vi "test_GetName.vi"() -> ()   [LabVIEW 2013]
uses:
  <vilib>/Utility/GetType.llb/Type Enum.ctl
  source/TypeDescriptor/TypeDescriptor_GetPString.vi
panel:
  out "Renamed Successfully":bool
  out "type descriptor dup 2":i16[](array[numeric]) format="%.0x"
  out "Type Enum 2":T1=enum."String"
  out "data string":string
  out "name":string
  out "interleaved array":u8[](array[numeric]) format="%.0x"
  out "type descriptor dup":i16[](array[numeric])
  # "index 2 = nb elements"
  # "size = 10 (xA)"
  # "Event DataType (x3 = I32)"
  # "size"
  # "TypeLabel (test)"
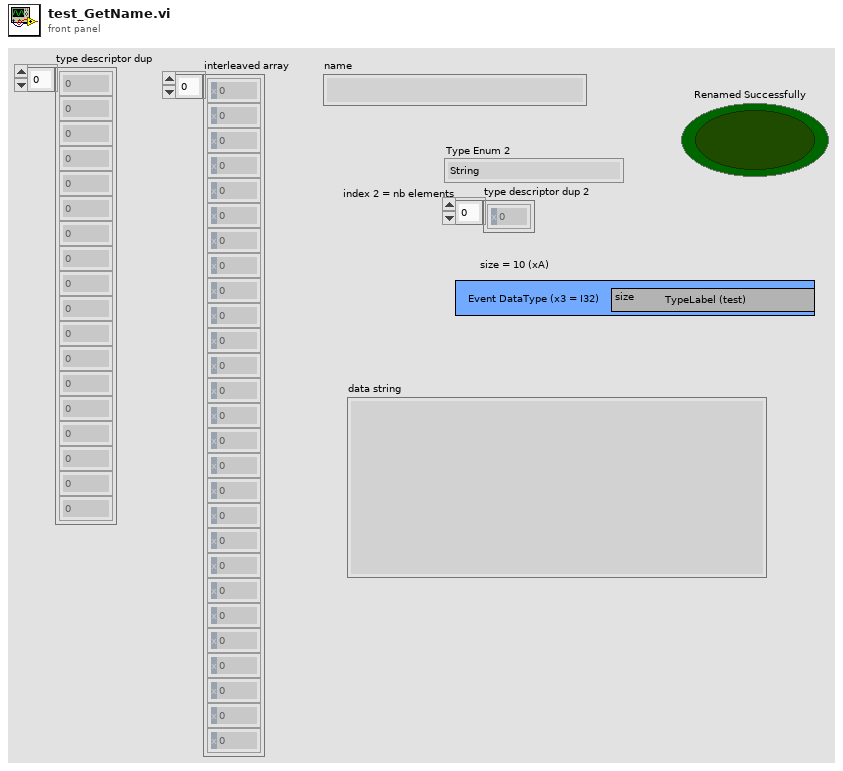
[diagram p1: front panel]
types:
  T1 = typedef "Type Enum.ctl" = enum8{"Void", "I8", "I16", "I32", "I64", "U8", "U16", "U32", "U64", "Single Float", "Double Float", "Extended Float", "Single Complex", "Double Complex", "Extended Complex", "Enum I8 NEVER", "Enum I16 NEVER", "Enum I32 NEVER", "Enum I64 NEVER", "Enum U8", "Enum U16", "Enum U32", "Enum U64", "Single Float With Unit", "Double Float With Unit", "Extended Float With Unit", "Single Complex With Unit", "Double Complex With Unit", "Extended Complex With Unit", "boolU16", "Boolean", "String", "Handle", "Path", "Picture", "C String", "Pascal String", "Tag", "SubString", "Array", "SubArray", "Cluster", "Numeric Cluster", "Variant", "LV Variant", "Measure Data (waveform)", "Refnum", "ExtData", "function", "Typedef", "Poly VI", "bad wire", "LabVIEW Class Instance"}
  T2 = typedef "Semaphore RefNum" = refnum<k1>
  T3 = cluster{"This is the boolean item's name":bool, "BBB":i32, "CCCC":string, "Data":dbl}
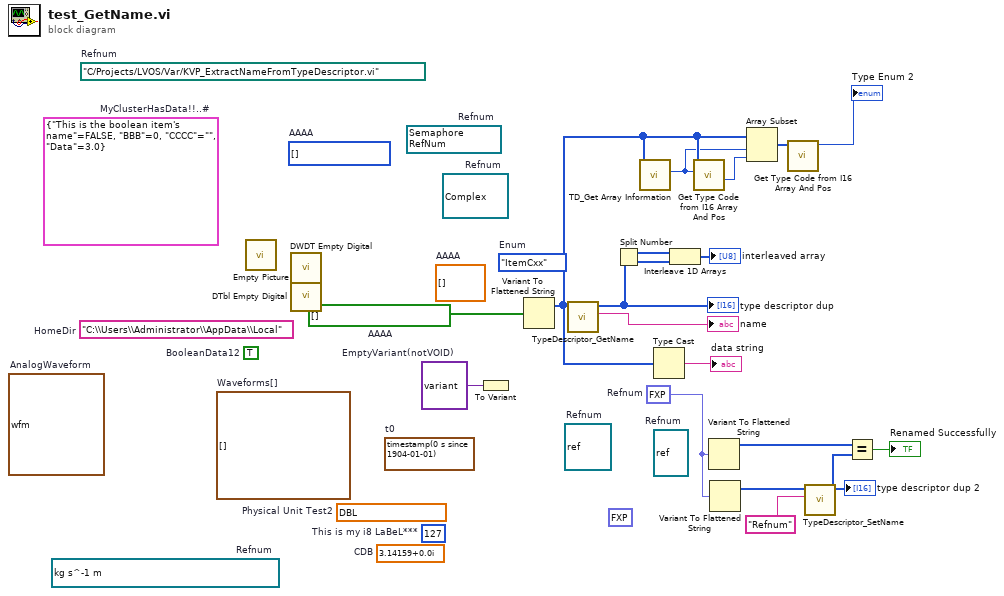
[diagram p0: block diagram]
diagram:
  (unwired) fxp<+,7,7> 127.0
  w1 = fxp<+,7,7> 127.0  # Refnum
  (unwired) refnum<class> refnum  # Refnum
  w14 = variant  # EmptyVariant(notVOID)
  (unwired) timestamp(0 s since 1904-01-01)  # t0
  (unwired) waveform(dbl)[] []  # Waveforms[]
  w8 = bool[] []  # AAAA
  (unwired) refnum<notifier> refnum items=["Item1", "Item2", "Item3A"]  # Refnum
  (unwired) T2 refnum items=["semaphore"]  # Refnum
  (unwired) refnum<queue> refnum  # Refnum
  (unwired) refnum<vi> refnum  # Refnum
  (unwired) waveform(dbl) {"t0"=timestamp(0 s since 1904-01-01), "dt"=1.0, "Y"=[]}  # AnalogWaveform
  (unwired) dbl[][] []  # AAAA
  (unwired) enum8{"Item1", "Item2", "Item3A"}[] [] items=["Item1", "Item2", "Item3A"]  # AAAA
  (unwired) cxt[unit] 3.141590118408203+0.0i  # Physical Unit Test2
  (unwired) path "C:/Projects/LVOS/Var/KVP_ExtractNameFromTypeDescriptor.vi"  # Refnum
  (unwired) T3 {"This is the boolean item's name"=FALSE, "BBB"=0, "CCCC"="", "Data"=3.0}  # MyClusterHasData!!..#
  (unwired) enum8{"A", "B2\ntest", "ItemCxx"}."ItemCxx"  # Enum
  (unwired) "C:\\Users\\Administrator\\AppData\\Local"  # HomeDir
  (unwired) TRUE  # BooleanData12
  (unwired) i8 127  # This is my i8 LaBeL***
  (unwired) cdb 3.14159+0.0i  # CDB
  n1 = call "Empty Picture"() -> ()  [unwired: 1 out]
  n2 = call <vilib>:"DWDT Empty Digital.vi"() -> ()  [unwired: 5 in, 1 out]
  n3 = call <vilib>:"DTbl Empty Digital.vi"() -> ()  [unwired: 5 in, 1 out]
  n4 = To Variant(anything=w14) -> ()  [unwired: 1 out]
  n5 = Variant To Flattened String(Variant=w8) -> (1:w12:i16[])  [unwired: 1 out]
  n6 = call "TypeDescriptor_GetName.vi"("type descriptor"=w12) -> ("name"=→"name":string, "type descriptor dup"=w17:i16[])  [unwired: 8 in, 1 out]
  "type descriptor dup" <- w17
  n7 = Split Number(x=w17) -> (hi(x)=w19:u8[], lo(x)=w18:u8[])
  n8 = call <vilib>:"TD_Get Array Information.vi"("Type descriptor"=w12) -> ("Contained TD Offset"=w11:i32)  [unwired: 8 in, 2 out]
  n9 = Type Cast(x=w12) -> (*(type *) &x=→"data string":string)  [unwired: 1 in]
  n10 = Interleave 1D Arrays(w19, w18) -> (→"interleaved array":u8[])
  n11 = call <vilib>:"Get Type Code from I16 Array And Pos.vi"("Pos in Type Descriptor (0)"=w11, "Type descriptor"=w12) -> ("Size (Words)"=w10:i32)  [unwired: 7 in, 2 out]
  n12 = Variant To Flattened String(Variant=w1) -> (1:w4:i16[])  [unwired: 1 out]
  n13 = Variant To Flattened String(Variant=w1) -> (1:w6:i16[])  [unwired: 1 out]
  n14 = Array Subset(array=w12, index=w11, length=w10) -> (w7:i16[])
  n15 = call <vilib>:"Get Type Code from I16 Array And Pos.vi"("Type descriptor"=w7) -> ("Type Enum"=→"Type Enum 2":T1)  [unwired: 8 in, 2 out]
  n16 = call "TypeDescriptor_SetName.vi"("name"="Refnum", "type descriptor"=w6) -> ("type descriptor dup"=w3:i16[])  [unwired: 7 in, 2 out]
  "type descriptor dup 2" <- w3
  n17 = Equal?(x=w4, y=w3) -> (x = y?=→"Renamed Successfully":bool)
